vi "Display Image.vi"(8 "error in (no error)":errorcluster, 11 "Frame Grabber Data in":T2={"Camera Session"="", "Frame"=refnum, "AVI Refnum"=refnum, "Codecs"=[], "Frame number"=0, "Tracking File Refnum"=refnum, "Tick Count"=0, "Probe Object"=refnum, "Playback Probe Data"=[], "Rigid Body"={"Position"={"x (mm)"=0.0, "y (mm)"=0.0, "z (mm)"=0.0}, "Orientation"={"Pitch (rad)"=0.0, "Yaw (rad)"=0.0, "Roll (rad)"=0.0}, "Quaternion"={"qx"=0.0, "qy"=0.0, "qz"=0.0, "qw"=0.0}, "Tracked?"=FALSE}, "Total no frames playback"=0, "Video FPS"=0.0, "Camera connected?"=FALSE, "Scene"=refnum, "Cropped Frame"=refnum, "Tracker FPS"=0.0, "Crop ROI"=[], "Presentation Values"=[], "Elapsed time (ms)"=0, "Camera frames playback"=0, "Refnums"={"Live Refnum"=refnum, "Record Refnum"=refnum, "Playback Refnum"=refnum, "Frame Slider Refnum"=refnum, "Pause Refnum"=refnum, "Home Refnum"=refnum, "Set Crop Refnum"=refnum, "Clear Crop Refnum"=refnum, "stop refnum"=refnum, "Playback Rate Refnum"=refnum, "Presentation Refnum"=refnum, "Crop Time Frame Slider Refnum"=refnum, "Cancel Save Refnum"=refnum, "Reverse Playback Refnum"=refnum, "Recording Settings Refnum"=refnum, "Continuous Playback Refnum"=refnum, "Annotation Refnum"=refnum, "Export All Refnum"=refnum, "Export List Refnum"=refnum, "Fill List Refnum"=refnum, "Save Crop Refnum"=refnum, "Skip Forward Refnum"=refnum, "Skip Backward Refnum"=refnum, "Single Annotation Refnum"=refnum, "Load Video Refnum"=refnum, "Set Start Refnum"=refnum, "Set End Refnum"=refnum, "Add to List Refnum"=refnum, "List of Annotations Refnum"=refnum, "Camera Frame Refnum"=refnum, "Load Image Refnum"=refnum, "Saving Refnum"=refnum}, "Dimensions"={"Probe Dimensions"={"Probe Width"=0.0, "Probe Depth"=1.0, "Probe Height"=0.0}, "Room Dimensions"={"Room Width"=0.0, "Room Depth"=0.0, "Room Height"=0.0}}, "Playback Data As Strings"=[], "Cropped Tracking File Refnum"=refnum, "Cropped AVI Refnum"=refnum, "Header"=[], "Total euclidian distance"=0.0, "Annotation File Path"=path "", "Playback File Path"=path "", "Size per frame"=0.0, "Ground Truth File Refnum"=refnum, "Annotation Array"=[], "Annotation TIFFs Folder"=path "", "overwriting open file?"=FALSE, "Image Sequence"=[], "Video/Image Flag"=enum."Playback Video Frame", "Image sequence?"=FALSE, "Image sequence filenames"=[], "Mask"=refnum}) -> (0 "error out":errorcluster, 1 "Continue playback?":bool, 2 "Image":T1, 3 "Frame Grabber Data out":T2={"Camera Session"="", "Frame"=refnum, "AVI Refnum"=refnum, "Codecs"=[], "Frame number"=0, "Tracking File Refnum"=refnum, "Tick Count"=0, "Probe Object"=refnum, "Playback Probe Data"=[], "Rigid Body"={"Position"={"x (mm)"=0.0, "y (mm)"=0.0, "z (mm)"=0.0}, "Orientation"={"Pitch (rad)"=0.0, "Yaw (rad)"=0.0, "Roll (rad)"=0.0}, "Quaternion"={"qx"=0.0, "qy"=0.0, "qz"=0.0, "qw"=0.0}, "Tracked?"=FALSE}, "Total no frames playback"=0, "Video FPS"=0.0, "Camera connected?"=FALSE, "Scene"=refnum, "Cropped Frame"=refnum, "Tracker FPS"=0.0, "Crop ROI"=[], "Presentation Values"=[], "Elapsed time (ms)"=0, "Camera frames playback"=0, "Refnums"={"Live Refnum"=refnum, "Record Refnum"=refnum, "Playback Refnum"=refnum, "Frame Slider Refnum"=refnum, "Pause Refnum"=refnum, "Home Refnum"=refnum, "Set Crop Refnum"=refnum, "Clear Crop Refnum"=refnum, "stop refnum"=refnum, "Playback Rate Refnum"=refnum, "Presentation Refnum"=refnum, "Crop Time Frame Slider Refnum"=refnum, "Cancel Save Refnum"=refnum, "Reverse Playback Refnum"=refnum, "Recording Settings Refnum"=refnum, "Continuous Playback Refnum"=refnum, "Annotation Refnum"=refnum, "Export All Refnum"=refnum, "Export List Refnum"=refnum, "Fill List Refnum"=refnum, "Save Crop Refnum"=refnum, "Skip Forward Refnum"=refnum, "Skip Backward Refnum"=refnum, "Single Annotation Refnum"=refnum, "Load Video Refnum"=refnum, "Set Start Refnum"=refnum, "Set End Refnum"=refnum, "Add to List Refnum"=refnum, "List of Annotations Refnum"=refnum, "Camera Frame Refnum"=refnum, "Load Image Refnum"=refnum, "Saving Refnum"=refnum}, "Dimensions"={"Probe Dimensions"={"Probe Width"=0.0, "Probe Depth"=1.0, "Probe Height"=0.0}, "Room Dimensions"={"Room Width"=0.0, "Room Depth"=0.0, "Room Height"=0.0}}, "Playback Data As Strings"=[], "Cropped Tracking File Refnum"=refnum, "Cropped AVI Refnum"=refnum, "Header"=[], "Total euclidian distance"=0.0, "Annotation File Path"=path "", "Playback File Path"=path "", "Size per frame"=0.0, "Ground Truth File Refnum"=refnum, "Annotation Array"=[], "Annotation TIFFs Folder"=path "", "overwriting open file?"=FALSE, "Image Sequence"=[], "Video/Image Flag"=enum."Playback Video Frame", "Image sequence?"=FALSE, "Image sequence filenames"=[], "Mask"=refnum}, 5 "Camera frame number":i32)   [LabVIEW 2017]
uses:
  Controls/Frame Grabber Data.ctl
  <vilib>/userdefined/High Color/IMAQdx.ctl
  <vilib>/vision/Image Controls.llb/IMAQ Image.ctl
  <vilib>/vision/Avi.llb/IMAQ AVI2 Refnum.ctl
  Controls/Rigid Body Info.ctl
  Controls/Position.ctl
  Controls/Orientation.ctl
  Controls/Refnums.ctl
  Controls/Recording Settings.ctl
  Controls/Operator Settings.ctl
  Controls/Operator.ctl
  Controls/Patient Settings.ctl
  Controls/Dimensions.ctl
  Controls/Room Dimensions.ctl
  Controls/Crop Video State.ctl
  <vilib>/vision/NI_Vision_Development_Module.lvlib
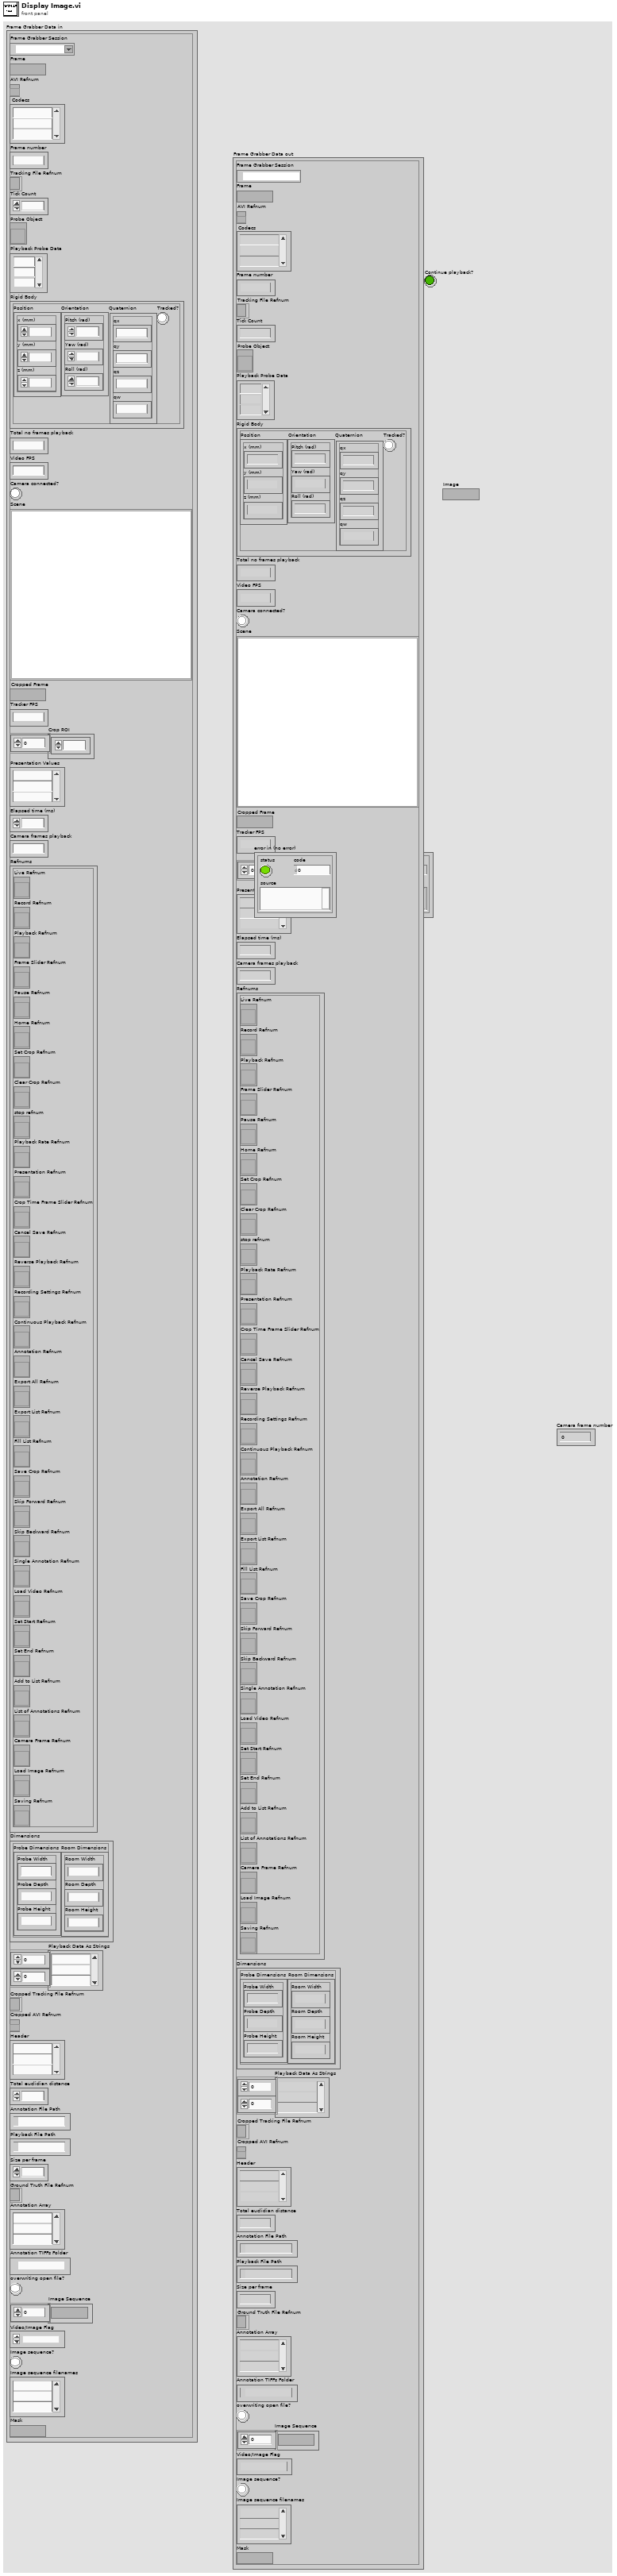
[diagram p1: front panel]
types:
  T1 = typedef "IMAQ Image.ctl" = refnum<image>
  T2 = typedef "Frame Grabber Data.ctl" = cluster{"Camera Session":T3, "Frame":T1, "AVI Refnum":T4, "Codecs":string[], "Frame number":u32, "Tracking File Refnum":refnum<file>, "Tick Count":u32, "Probe Object":refnum<vi>, "Playback Probe Data":dbl[][], "Rigid Body":T5, "Total no frames playback":i32, "Video FPS":dbl, "Camera connected?":bool, "Scene":refnum<vi>, "Cropped Frame":T1, "Tracker FPS":dbl, "Crop ROI":i32[], "Presentation Values":string[], "Elapsed time (ms)":u32, "Camera frames playback":u32, "Refnums":T8, "Dimensions":T9, "Playback Data As Strings":string[][], "Cropped Tracking File Refnum":refnum<file>, "Cropped AVI Refnum":T4, "Header":string[], "Total euclidian distance":dbl, "Annotation File Path":path, "Playback File Path":path, "Size per frame":dbl, "Ground Truth File Refnum":refnum<file>, "Annotation Array":string[], "Annotation TIFFs Folder":path, "overwriting open file?":bool, "Image Sequence":T1[], "Video/Image Flag":T11, "Image sequence?":bool, "Image sequence filenames":string[], "Mask":T1}
  T3 = typedef "IMAQdx.ctl" = refnum<k21>
  T4 = typedef "IMAQ AVI2 Refnum.ctl" = refnum<k20>
  T5 = typedef "Rigid Body Info.ctl" = cluster{"Position":T6, "Orientation":T7, "Quaternion":cluster{"qx":sgl, "qy":sgl, "qz":sgl, "qw":sgl}, "Tracked?":bool}
  T6 = typedef "Position.ctl" = cluster{"x (mm)":sgl, "y (mm)":sgl, "z (mm)":sgl}
  T7 = typedef "Orientation.ctl" = cluster{"Pitch (rad)":sgl, "Yaw (rad)":sgl, "Roll (rad)":sgl}
  T8 = typedef "Refnums.ctl" = cluster{"Live Refnum":refnum<vi>, "Record Refnum":refnum<vi>, "Playback Refnum":refnum<vi>, "Frame Slider Refnum":refnum<vi>, "Pause Refnum":refnum<vi>, "Home Refnum":refnum<vi>, "Set Crop Refnum":refnum<vi>, "Clear Crop Refnum":refnum<vi>, "stop refnum":refnum<vi>, "Playback Rate Refnum":refnum<vi>, "Presentation Refnum":refnum<vi>, "Crop Time Frame Slider Refnum":refnum<vi>, "Cancel Save Refnum":refnum<vi>, "Reverse Playback Refnum":refnum<vi>, "Recording Settings Refnum":refnum<vi>, "Continuous Playback Refnum":refnum<vi>, "Annotation Refnum":refnum<vi>, "Export All Refnum":refnum<vi>, "Export List Refnum":refnum<vi>, "Fill List Refnum":refnum<vi>, "Save Crop Refnum":refnum<vi>, "Skip Forward Refnum":refnum<vi>, "Skip Backward Refnum":refnum<vi>, "Single Annotation Refnum":refnum<vi>, "Load Video Refnum":refnum<vi>, "Set Start Refnum":refnum<vi>, "Set End Refnum":refnum<vi>, "Add to List Refnum":refnum<vi>, "List of Annotations Refnum":refnum<vi>, "Camera Frame Refnum":refnum<vi>, "Load Image Refnum":refnum<vi>, "Saving Refnum":refnum<vi>}
  T9 = typedef "Dimensions.ctl" = cluster{"Probe Dimensions":cluster{"Probe Width":sgl, "Probe Depth":sgl, "Probe Height":sgl}, "Room Dimensions":T10}
  T10 = typedef "Room Dimensions.ctl" = cluster{"Room Width":dbl, "Room Depth":dbl, "Room Height":dbl}
  T11 = typedef "Crop Video State.ctl" = enum16{"Init", "Wait", "Load Image", "Load Video", "Play/Pause", "Playback Video Frame", "Display Image", "Save Image Sequence", "Save Video", "Export List", "Export All", "Close", "Set Crop Area", "Reset Crop Area", "Crop Inside", "Crop Outside", "Multi-Crop", "Re-Open Files", "Annotate Frame", "Annotate Clip", "Add to List", "Fill List", "Set Start", "Set End", "Error Handling", "Shutdown"}
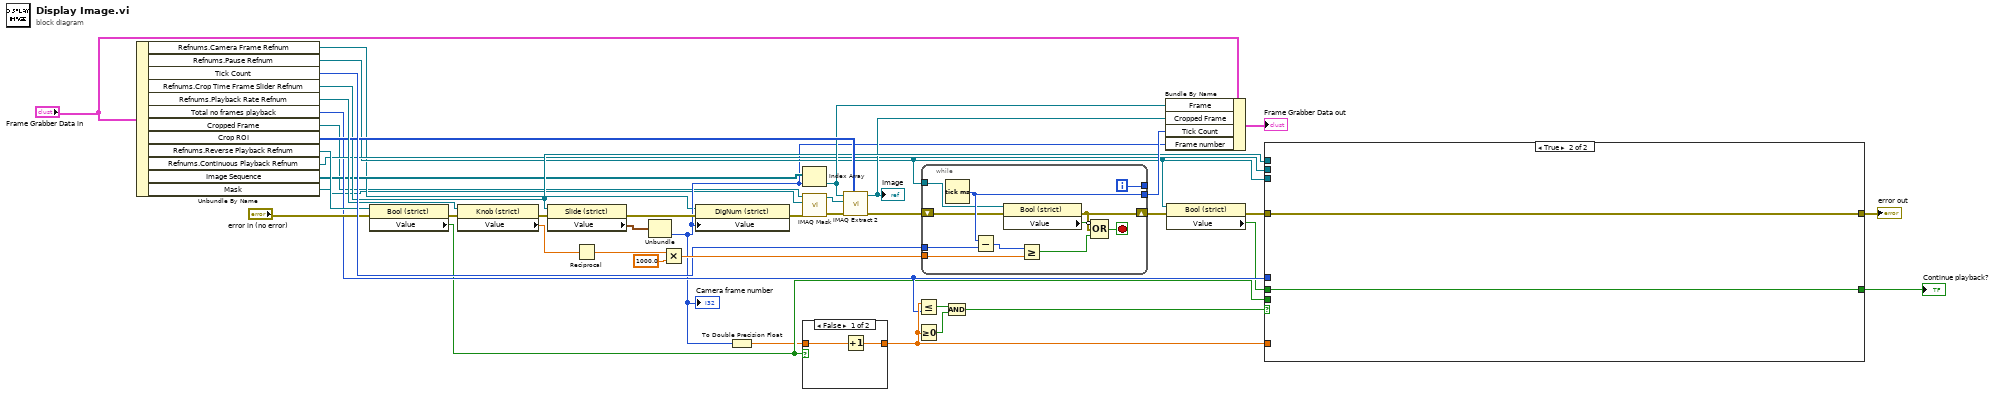
[diagram p0: block diagram]
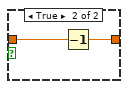
[diagram p2: hidden frame]
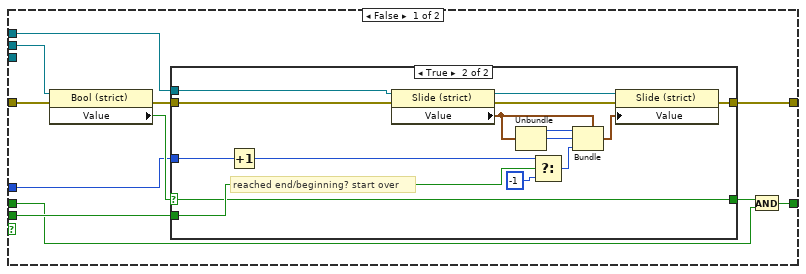
[diagram p3: hidden frame]
diagram:
  n1 = Unbundle By Name("Frame Grabber Data in") -> ("Refnums.Camera Frame Refnum"=w6:refnum<vi>, "Refnums.Pause Refnum"=w12:refnum<vi>, "Tick Count"=w37:u32, "Refnums.Crop Time Frame Slider Refnum"=w27:refnum<vi>, "Refnums.Playback Rate Refnum"=w33:refnum<vi>, "Total no frames playback"=w17:i32, "Cropped Frame"=w2:T1, "Crop ROI"=w29:i32[], "Refnums.Reverse Playback Refnum"=w23:refnum<vi>, "Refnums.Continuous Playback Refnum"=w18:refnum<vi>, "Image Sequence"=w8:T1[], "Mask"=w3:T1)
  n2 = property class="Bool (strict)"(reference=w23, error in="error in (no error)") -> (error out=w24:errorcluster, "Value"=w16:bool)  [unwired: 1 out]
  n3 = property class="Knob (strict)"(reference=w33, error in=w24) -> (error out=w34:errorcluster, "Value"=w35:dbl)  [unwired: 1 out]
  n4 = property class="Slide (strict)"(reference=w27, error in=w34) -> (error out=w14:errorcluster, "Value"=w32:cluster{i32, i32, i32})  [unwired: 1 out]
  n5 = Reciprocal(x=w35) -> (1/x=w40:dbl)
  n6 = Unbundle(w32) -> (w7:i32)  [unwired: 2 out]
  "Camera frame number" <- w7
  n7 = Multiply(x=w40, y=1000.0) -> (x*y=w38:dbl)
  n8 = property class="DigNum (strict)"(reference=w6, error in=w14, "Value"=w7) -> (error out=w5:errorcluster)  [unwired: 1 out]
  n9 = To Double Precision Float(number=w7) -> (double precision float=w13:dbl)
  n10 = Index Array(array=w8, index=w7) -> (element=w28:T1)
  n11 = call "IMAQ Mask"("error in (no error)"=w5, "Image Mask"=w3, "Image Src"=w2) -> ("error out"=w4:errorcluster, "Image Dst Out"=w1:T1)  [unwired: 2 in]
  n12 = case shown="False" w16 {
    tunnel: [w44 w45] -> w21
    tunnel: w13 -> [w43 w46]
    frame False {
      n13 = Increment(x=w43) -> (x+1=w44:dbl)
    }
    frame True {
      n14 = Decrement(x=w46) -> (x-1=w45:dbl)
    }
  }
  n15 = call "IMAQ Extract 2"("Optional Rectangle"=w29, "error in (no error)"=w4, "Image Dst"=w1, "Image Src"=w28) -> ("error out"=w36:errorcluster, "Image Dst Out"=w20:T1)  [unwired: 6 in]
  "Image" <- w20
  n16 = Less Or Equal?(x=w21, y=w17) -> (x <= y?=w30:bool)
  n17 = Greater Or Equal To 0?(x=w21) -> (x >= 0?=w22:bool)
  n18 = while {
    tunnel: [w57] -> w41
    tunnel: w38 -> [w55]
    tunnel: w37 -> [w54]
    shift-right: [w50] -> w11
    shift-left: w36 -> [w51]
    tunnel: w12 -> [w49]
    tunnel: [w47] -> _
    i -> [w47]
    stop <- w53 stop-if-true
    n19 = Tick Count (ms)() -> (millisecond timer value=w57:u32)
    n20 = Subtract(x=w57, y=w54) -> (x-y=w56:u32)
    n21 = property class="Bool (strict)"(reference=w49, error in=w51) -> (error out=w50:errorcluster, "Value"=w48:bool)  [unwired: 1 out]
    n22 = Greater Or Equal?(x=w56, y=w55) -> (x >= y?=w52:bool)
    n23 = Compound Arithmetic op=OR(invert w48, w50, w52) -> (w53:bool)
  }
  n24 = And(x=w30, y=w22) -> (x .and. y?=w26:bool)
  n25 = Bundle By Name(cluster="Frame Grabber Data in", "Frame"=w28, "Cropped Frame"=w20, "Tick Count"=w41, "Frame number"=w7) -> (→"Frame Grabber Data out":T2)
  n26 = property class="Bool (strict)"(reference=w12, error in=w11) -> (error out=w10:errorcluster, "Value"=w9:bool)  [unwired: 1 out]
  n27 = case shown="True" w26 {
    tunnel: w10 -> [w65 w87]
    tunnel: w12 -> [_ _]
    tunnel: w21 -> [_ _]
    tunnel: w27 -> [w68 _]
    tunnel: [w67 w87] -> w19
    tunnel: w18 -> [w66 _]
    tunnel: w17 -> [w62 _]
    tunnel: w16 -> [w61 _]
    tunnel: [w59 w86] -> w15
    tunnel: w9 -> [w58 w86]
    frame False {
      n28 = property class="Bool (strict)"(reference=w66, error in=w65) -> (error out=w64:errorcluster, "Value"=w63:bool)  [unwired: 1 out]
      n29 = case shown="True" w63 {
        selector: w63 -> [w69 w73]
        tunnel: w68 -> [_ w85]
        tunnel: [w70 w84] -> w67
        tunnel: w64 -> [w70 w83]
        tunnel: w62 -> [_ w75]
        tunnel: w61 -> [_ w74]
        tunnel: [w69 w73] -> w60
        frame False {
        }
        frame True {
          # "reached end/beginning? start over"
          n30 = Increment(x=w75) -> (x+1=w71:i32)
          n31 = property class="Slide (strict)"(reference=w85, error in=w83) -> (reference out=w82:refnum<vi>, error out=w78:errorcluster, "Value"=w72:cluster{i32, i32, i32})
          n32 = Unbundle(w72) -> (w79:i32, w80:i32)  [unwired: 1 out]
          n33 = Select(t=w71, s=w74, f=-1) -> (s? t:f=w76:i32)
          n34 = Bundle(cluster=w72, w79, w80, w76) -> (w81:cluster{i32, i32, i32})
          n35 = property class="Slide (strict)"(reference=w82, error in=w78, "Value"=w81) -> (error out=w84:errorcluster)  [unwired: 1 out]
        }
      }
      n36 = And(x=w60, y=w58) -> (x .and. y?=w59:bool)
    }
    frame True {
    }
  }
  "error out" <- w19
  "Continue playback?" <- w15
